vi "Timing Loop.vi"(5 "VolatusAPI":refnum<class "VolatusAPI.lvclass">, 6 "Seq Name":string, 7 "Period":i64, 9 "Loop Data in":T1, 11 "Sequence in":refnum<class "Sequence.lvclass">) -> (1 "Loop Data":T1)   [LabVIEW 2023, in "VolatusSeq.lvlib" / "Sequence.lvclass"]
uses:
  Sequence.lvclass
  Loop Data.ctl
  Volatus/MessageQ/MessageQ.lvclass
  Sequence Time.ctl
  Volatus/VolatusAPI/VolatusAPI.lvclass
  <vilib>/Platform/TimedLoop/XDataNode/timing_clust.ctl
  <vilib>/Platform/TimedLoop/XDataNode/nitl_modes.ctl
  <vilib>/Platform/TimedLoop/XDataNode/wakeup.ctl
  Sequence.lvclass/Sequence.ctl
  <vilib>/platform/TimedLoop/XDataNode/XDataNode.xnode
  <vilib>/Platform/TimedLoop/XDataNode/XDNodeRunTimeDep.lvlib
  State/State.lvclass
  VolatusSeq.lvlib
  VolatusSeqConfig/Debug Flags.ctl
  VolatusSeqConfig/VolatusSeqConfig.lvlib
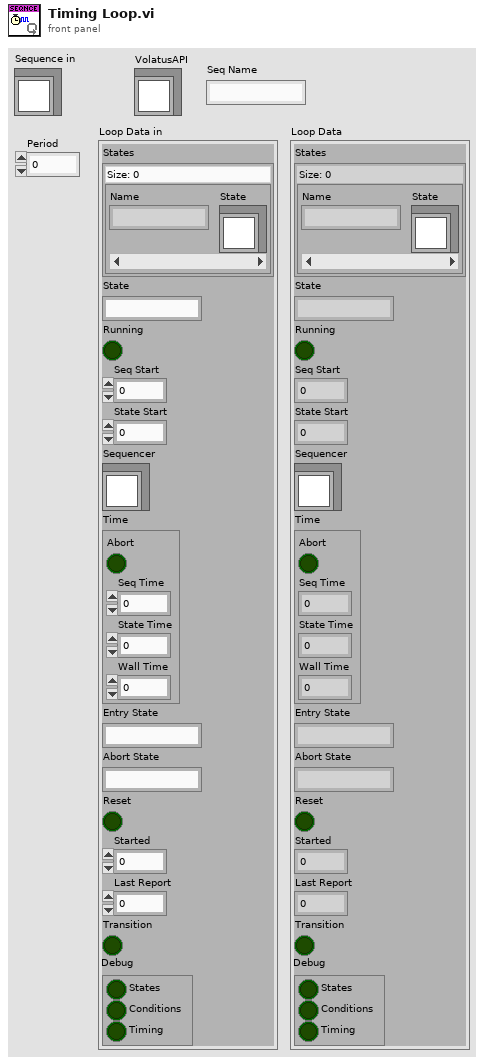
[diagram p1: front panel]
types:
  T1 = typedef "VolatusSeq.lvlib/Sequence.lvclass/Loop Data.ctl" = cluster{"States":map{string, refnum<class "State.lvclass">}, "State":string, "Running":bool, "Seq Start":dbl, "State Start":dbl, "Sequencer":refnum<class "MessageQ.lvclass">, "Time":T2, "Entry State":string, "Abort State":string, "Reset":bool, "Started":dbl, "Last Report":dbl, "Transition":bool, "Debug":T3}
  T2 = typedef "VolatusSeq.lvlib/Sequence Time.ctl" = cluster{"Abort":bool, "Seq Time":dbl, "State Time":dbl, "Wall Time":dbl}
  T3 = typedef "VolatusSeqConfig.lvlib/Debug Flags.ctl" = cluster{"States":bool, "Conditions":bool, "Timing":bool}
  T4 = typedef "XDNodeRunTimeDep.lvlib/timing_clust.ctl" = cluster{"Expected End [f-1]":u64, "Actual End [f-1]":u64, "Finished Late? [f-1]":bool, "Expected End [i-1]":u64, "Actual End [i-1]":u64, "Finished Late? [i-1]":bool, "Expected Start [i]":u64, "Actual Start [i]":u64, "Expected Start [f]":u64, "Actual Start [f]":u64, "Source Name":string, "Structure Name":string, "Period":i64, "Deadline":i64, "Offset":i64, "Start":i64, "Priority":i32, "Timeout":i32, "Mode":T5, "Wakeup Reason":T6, "Error":errorcluster, "Source Type":string, "Secondary Source Type":string, "Global End Time":u64, "Global Start Time":u64, "Frame Duration":u64, "Iteration Duration":u64, "Assigned CPU":i32, "I/O Scan Engine Mode":u32}
  T5 = typedef "XDNodeRunTimeDep.lvlib/nitl_modes.ctl" = enum32{"No Change", "Process missed periods, maintain original phase", "Discard missed periods, maintain original phase", "Process missed periods, ignore original phase", "Discard missed periods, ignore original phase"}
  T6 = typedef "XDNodeRunTimeDep.lvlib/wakeup.ctl" = enum32{"Normal", "Aborted", "Asynchronous wakeup", "Timing source error", "Timed loop error", "Timeout"}
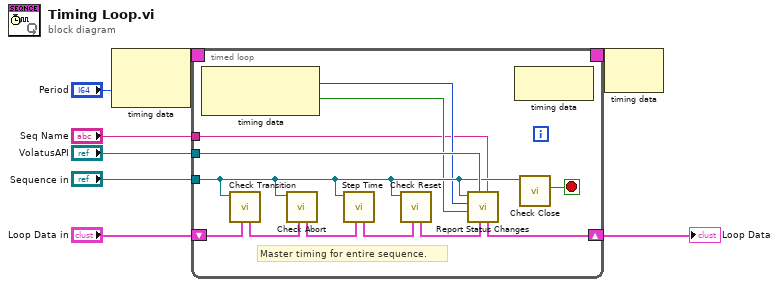
[diagram p0: block diagram]
diagram:
  n1 = node-c288("Period") -> (w4:T4)  [unwired: 1 in]
  n2 = timed-loop {
    shift-right: [w17] -> w5
    shift-left: "Loop Data in" -> [w20]
    tunnel: "Sequence in" -> [w14]
    tunnel: "VolatusAPI" -> [w18]
    timing: w4 -> [_]
    timing-out: [_] -> w3
    tunnel: "Seq Name" -> [w9]
    stop <- w19 stop-if-true
    # "Master timing for entire sequence."
    n3 = node-c288() -> (w11:i64, w10:bool)  [unwired: 1 in]
    n4 = call "Check Transition.vi"("Loop Data in"=w20, "Sequence in"=w14) -> ("Loop Data"=w13:T1)  [unwired: 9 in]
    n5 = call "Check Abort.vi"("Loop Data in"=w13, "Sequence in"=w14) -> ("Loop Data"=w12:T1)  [unwired: 9 in]
    n6 = call "Step Time.vi"("Loop Data in"=w12, "Sequence in"=w14) -> ("Loop Data"=w16:T1)  [unwired: 9 in]
    n7 = call "Check Reset.vi"("Loop Data in"=w16, "Sequence in"=w14) -> ("Loop Data"=w15:T1)  [unwired: 9 in]
    n8 = call "Report Status Changes.vi"("Seq Name"=w9, "Loop Data in"=w15, "VolatusAPI"=w18, "Previous Late"=w10, "Previous Duration"=w11, "Sequence in"=w14) -> ("Loop Data"=w17:T1)  [unwired: 5 in]
    n9 = node-c288() -> ()  [unwired: 1 in, 1 out]
    n10 = call "Check Close.vi"("Sequence in"=w14) -> ("Close"=w19:bool)  [unwired: 10 in]
  }
  "Loop Data" <- w5
  n11 = node-c288(w3) -> ()  [unwired: 1 out]
